vi "Motor.Release.vi"(5 "Motor":T2 items=["Port A", "Port B", "Port C"], 7 "MotorBits":u8 format="%.0b", 10 "Cancelled?":bool) -> ()   [LabVIEW 2009]
uses:
  <vilib>/NXT/Block Support/NXT_OutputPort.ctl
  NXTOutputRefnum.ctl
  Move/RunState.ctl
  Program Files/National Instruments/LabVIEW 2009/resource/objmgr/NXTInputOutput.rc
panel:
  in  "Generic Refnum Name":T1
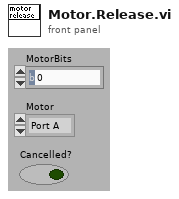
[diagram p1: front panel]
types:
  T1 = typedef "NXTOutputRefnum.ctl" = refnum<k21>
  T2 = typedef "NXT_OutputPort.ctl" = u8
  T3 = typedef "RunState.ctl" = u8
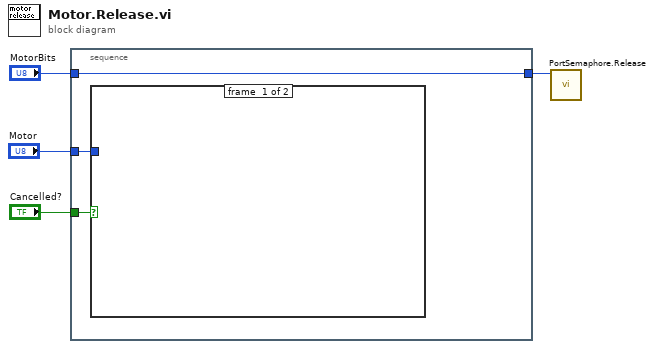
[diagram p0: block diagram]
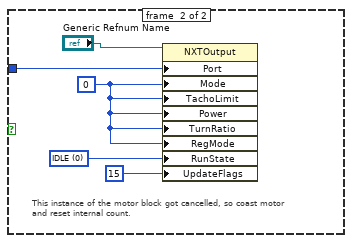
[diagram p2: hidden frame]
diagram:
  n1 = stacked-sequence {
    tunnel: "Cancelled?" -> [w7]
    tunnel: "Motor" -> [w6]
    tunnel: [w5] -> w3
    tunnel: "MotorBits" -> [w5]
    frame #0 {
      n2 = case shown="True" w7 {
        tunnel: w6 -> [_ w8]
        frame #0 {
        }
        frame #1 {
          w10 = u8 0 ("f")
          w11 = T3 0 items=["IDLE"=0, "RAMPUP"=16, "RUNNING"=32, "RAMPDOWN"=64] ("RunState")
          # "This instance of the motor block got cancelled, so coast motor\nand reset internal count."
          n3 = property class="NXTOutput"(reference="Generic Refnum Name", "Port"=w8, "Mode"=w10, "TachoLimit"=w10, "Power"=w10, "TurnRatio"=w10, "RegMode"=w10, "RunState"=w11, "UpdateFlags"=u8 15) -> ()  [unwired: 1 in, 2 out]
        }
      }
    }
  }
  n4 = call <vilib>:"PortSemaphore.Release.vi"("MotorBits"=w3) -> ()  [unwired: 11 in]
